vi "PlumeCenterDetermination.vi"(7 "nPointsSampled":i32, 10 "SD Estimate":dbl, 11 "nPointsInRake":i32) -> (2 "CommandString":string, 3 "Measurement Center":dbl)   [LabVIEW 2011]
uses:
  GaussianGlobal.vi
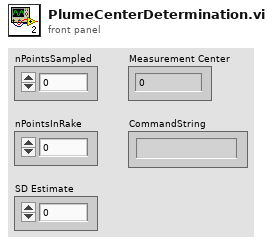
[diagram p1: front panel]
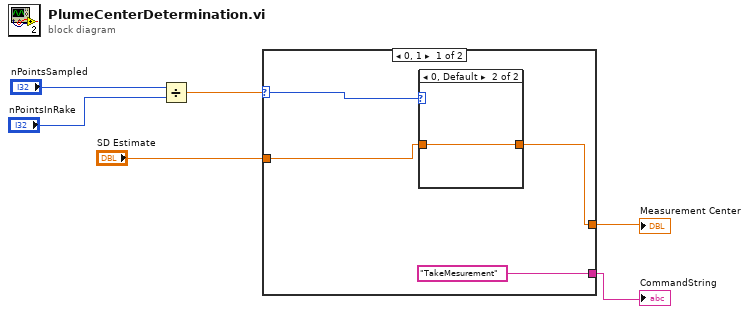
[diagram p0: block diagram]
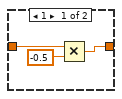
[diagram p2: hidden frame]
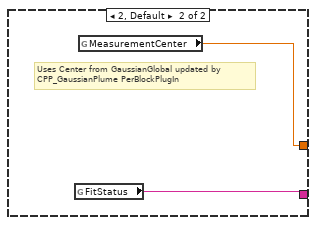
[diagram p3: hidden frame]
diagram:
  n1 = Divide(x="nPointsSampled", y="nPointsInRake") -> (x/y=w4:dbl)
  n2 = case shown="0, 1" w4 {
    selector: w4 -> [w10 _]
    tunnel: [w9 w16] -> w1
    tunnel: "SD Estimate" -> [w8 _]
    tunnel: ["TakeMesurement" w15] -> w6
    frame 0, 1 {
      n3 = case shown="0, Default" w10 {
        tunnel: w8 -> [w13 w14]
        tunnel: [w11 w14] -> w9
        frame 1 {
          n4 = Multiply(x=w13, y=-0.5) -> (x*y=w11:dbl)
        }
        frame 0, Default {
        }
      }
    }
    frame 2, Default {
      # "Uses Center from GaussianGlobal updated by\nCPP_GaussianPlume PerBlockPlugIn"
      n5 = global read "GaussianGlobal.vi" "FitStatus"() -> (w15:string)
      n6 = global read "GaussianGlobal.vi" "MeasurementCenter"() -> (w16:dbl)
    }
  }
  "CommandString" <- w6
  "Measurement Center" <- w1
